vi "Asylum_Driver_LithographyInitialize.vi"(8 "error in (no error)":errorcluster, 11 "Background Image":path=path "Q:/inst/AFM Drift/SAA00010002.ibw") -> (0 "error out":errorcluster, 3 "Offset out":cluster{"X":dbl, "Y":dbl})   [LabVIEW 2020]
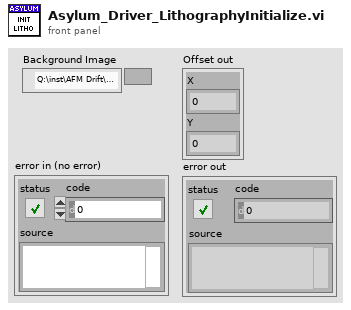
[diagram p1: front panel]
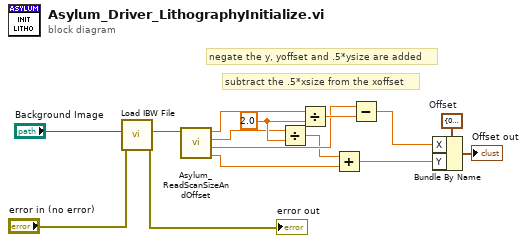
[diagram p0: block diagram]
diagram:
  w11 = 2.0
  w12 = cluster{"X":dbl, "Y":dbl} {"X"=0.0, "Y"=0.0}  # Offset
  # "subtract the .5*xsize from the xoffset"
  # "negate the y, yoffset and .5*ysize are added"
  n1 = call "Load IBW File.vi"("error in (no error)"="error in (no error)", "file path (dialog if empty)"="Background Image") -> ("error out"=→"error out":errorcluster, "Wave Note"=w15:string)  [unwired: 7 in, 1 out]
  n2 = call "Asylum_ReadScanSizeAndOffset.vi"("Read in the string file"=w15) -> ("Y Offset"=w5:dbl, "X Offset"=w8:dbl, "Y Range"=w9:dbl, "X Range"=w7:dbl)  [unwired: 7 in]
  n3 = Divide(x=w9, y=w11) -> (x/y=w6:dbl)
  n4 = Divide(x=w7, y=w11) -> (x/y=w10:dbl)
  n5 = Add(x=w6, y=w5) -> (x+y=w3:dbl)
  n6 = Subtract(x=w8, y=w10) -> (x-y=w4:dbl)
  n7 = Bundle By Name(cluster=w12, "X"=w4, "Y"=w3) -> (→"Offset out":cluster{"X":dbl, "Y":dbl})
